vi "Reshape 2D to 3D data.vi"(0 "Parameters In (2D)":cdb[][](array[numeric]) format="%.3f", 11 "Error In":errorcluster) -> (4 "Parameters Out (3D)":cdb[][][](array[numeric]) format="%.3f", 15 "Error Out":errorcluster)   [LabVIEW 2023, in "NI_HFNetworkAnalysis.lvlib"]
doc: "Transforms a 2D array of network parameters into a 3D array for matrix calculations.\n\nInput array element rows are assumed as \n <b>(x11,x12,x13,...,x21,x22,x23,...,x31,x32,x33,...)</b>\nand resulting 3D array pages are defined as\n <b>((x11,x12,x13,...),\n (x21,x22,x23,...),\n (x31,x32,x33,...),\n ...)</b>"
uses:
  NI_HFNetworkAnalysis.lvlib
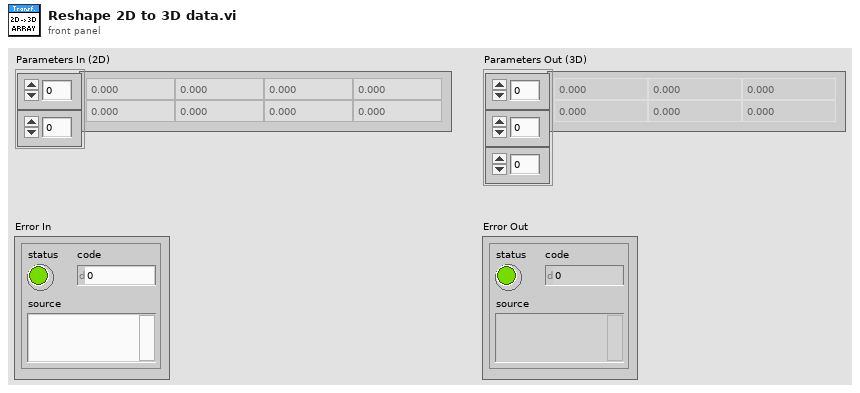
[diagram p1: front panel]
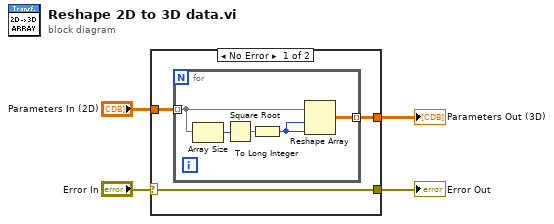
[diagram p0: block diagram]
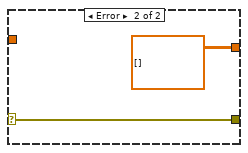
[diagram p2: hidden frame]
diagram:
  n1 = case shown="No Error" "Error In" {
    selector: "Error In" -> [w5 w13]
    tunnel: "Parameters In (2D)" -> [w7 _]
    tunnel: [w6 cdb[][][] []] -> w3
    tunnel: [w5 w13] -> w1
    frame No Error {
      n2 = for {
        tunnel: w7 -> [w10] mode=indexing
        tunnel: [w8] -> w6 mode=indexing
        n3 = Array Size(array=w10) -> (size(s)=w12:i32)
        n4 = Square Root(x=w12) -> (sqrt(x)=w11:dbl)
        n5 = To Long Integer(number=w11) -> (32bit integer=w9:i32)
        n6 = Reshape Array(w10, w9, w9) -> (w8:cdb[][])
      }
    }
    frame Error {
    }
  }
  "Parameters Out (3D)" <- w3
  "Error Out" <- w1
